vi "counter_sum.vi"(8 "error in":errorcluster) -> (0 "error IO":errorcluster, 1 "Number of Hours":dbl, 2 "Third Detector Sum":i64, 3 "First Detector Sum":i64)   [LabVIEW 2012]
uses:
  <vilib>/addons/database/Auxilliary.llb/DB Tools Parameter Info.ctl
  <vilib>/addons/database/Auxilliary.llb/DB Tools DataTypes.ctl
  <vilib>/addons/database/Auxilliary.llb/DB Tools Parameter Dir.ctl
  <vilib>/addons/database/Command.llb/Cmd Execute.vi
  <vilib>/addons/database/Recordset.llb/Rec Fetch Recordset Data (CR).vi
  <vilib>/addons/database/Recordset.llb/Rec Destroy - Command.vi
  <vilib>/addons/database/Command.llb/Cmd Delete.vi
  <vilib>/addons/database/Connection.llb/Conn Execute.vi
  <vilib>/addons/database/Recordset.llb/Rec Fetch Recordset Data (R).vi
  <vilib>/addons/database/Recordset.llb/Rec Destroy - Connection.vi
  <vilib>/addons/database/Command.llb/Cmd Set Parameter Value (C).vi
  <vilib>/addons/database/_DB Variant To Data/Database Variant To Data.xnode
  <vilib>/addons/database/NI_Database_API.lvlib
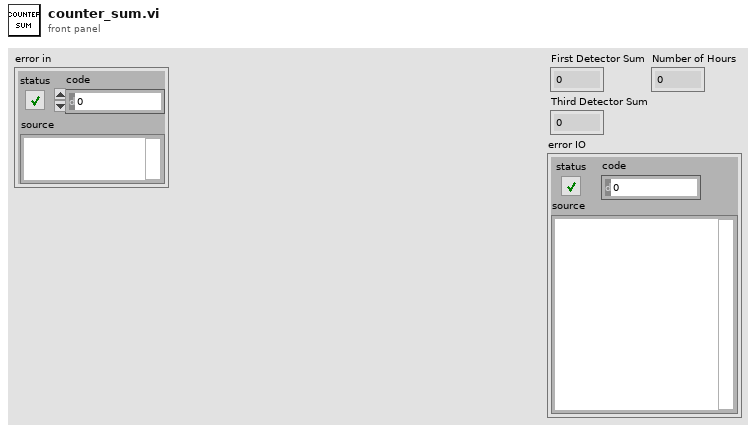
[diagram p1: front panel]
types:
  T1 = typedef "NI_Database_API.lvlib/DB Tools Parameter Info.ctl" = cluster{"parameter name":string, "type":T2, "direction":T3, "value":variant}
  T2 = typedef "NI_Database_API.lvlib/DB Tools DataTypes.ctl" = enum16{"String", "Long (I32)", "Single (SGL)", "Double (DBL)", "Date/Time", "Binary"}
  T3 = typedef "NI_Database_API.lvlib/DB Tools Parameter Dir.ctl" = enum32{"Input", "Output", "Input/Output", "Return Value"}
  T4 = typedef "NI_Database_API.lvlib/Conn ObjectReference.ctl" = refnum<k1>
  T5 = typedef "NI_Database_API.lvlib/Cmd ObjectReference.ctl" = refnum<k1>
  T6 = typedef "NI_Database_API.lvlib/Cmd-Rec Object Reference.ctl" = refnum<k1>
  T7 = typedef "NI_Database_API.lvlib/Rec ObjectReference.ctl" = refnum<k1>
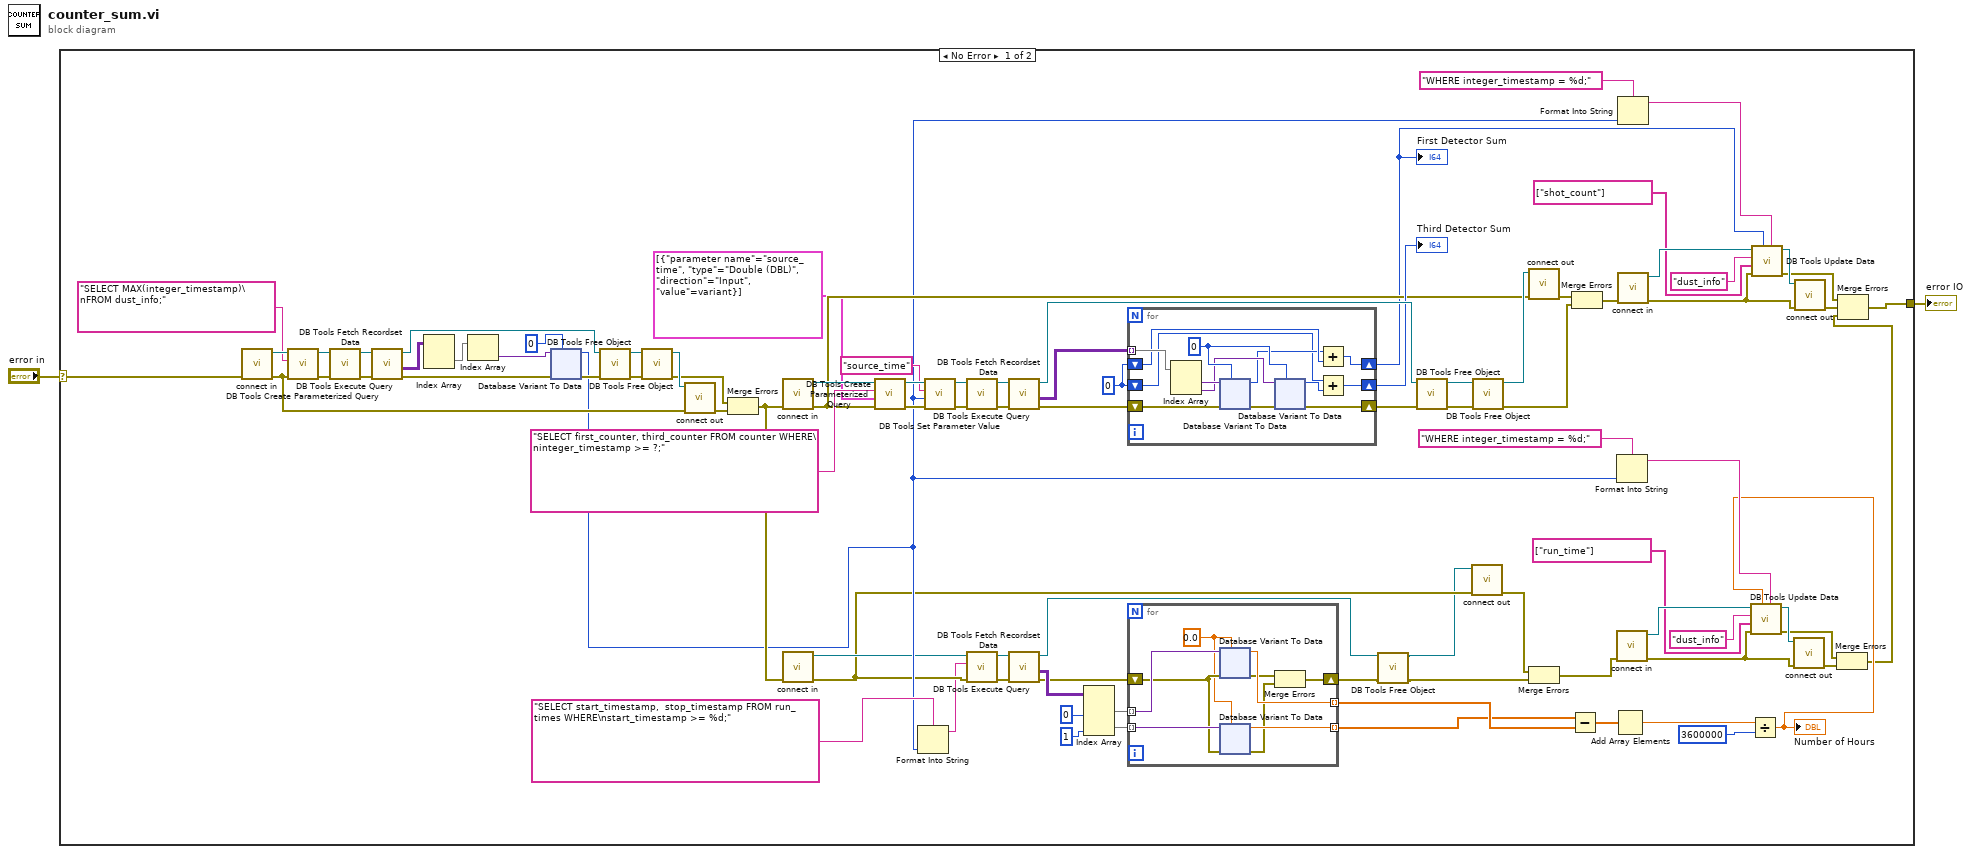
[diagram p0: block diagram]
diagram:
  n1 = case shown="No Error" "error in" {
    selector: "error in" -> [w92 w275]
    tunnel: [w49 w275] -> w1
    frame No Error {
      w60 = i64 0
      n2 = call "connect in.vi"("error in (no error)"=w92) -> ("error out"=w57:errorcluster, "Database Connection"=w91:T4)  [unwired: 6 in, 1 out]
      n3 = call <vilib>:"DB Tools Create Parameterized Query.vi"("error in (no error)"=w57, "SQL query"="SELECT MAX(integer_timestamp)\nFROM dust_info;", "connection reference"=w91) -> ("error out"=w88:errorcluster, "command reference"=w89:T5)  [unwired: 4 in, 1 out]
      n4 = call-poly <vilib>:"DB Tools Execute Query.vi"("error in (no error)"=w88, "command reference"=w89) -> ("error out"=w86:errorcluster, "command-recordset reference"=w87:T6)  [unwired: 6 in]
      n5 = call-poly <vilib>:"DB Tools Fetch Recordset Data.vi"("error in (no error)"=w86, "command-recordset reference"=w87) -> ("error out"=w78:errorcluster, "recordset data"=w82:variant[][], "command-recordset reference out"=w85:T6)  [unwired: 3 in]
      n6 = Index Array(array=w82) -> (element=w81:variant[])  [unwired: 2 in]
      n7 = Index Array(array=w81) -> (element=w80:variant)  [unwired: 1 in]
      n8 = xnode "Database Variant To Data"("database variant"=w80, "error in (no error)"=w78, "type"=i64 0) -> ("data"=w10:i64, "error out"=w77:errorcluster)
      n9 = call-poly <vilib>:"DB Tools Free Object.vi"("error in (no error)"=w77, "command-recordset reference"=w85) -> ("error out"=w83:errorcluster, "command reference"=w84:T5)  [unwired: 8 in]
      n10 = call-poly <vilib>:"DB Tools Free Object.vi"("error in (no error)"=w83, "command reference"=w84) -> ("error out"=w53:errorcluster, "connection reference"=w58:T4)  [unwired: 8 in]
      n11 = call "connect out.vi"("error in (no error)"=w57, "connection reference"=w58) -> ("error out"=w54:errorcluster)  [unwired: 9 in]
      n12 = Merge Errors(w53, w54) -> (w39:errorcluster)
      n13 = call "connect in.vi"("error in (no error)"=w39) -> ("error out"=w55:errorcluster, "Database Connection"=w56:T4)  [unwired: 6 in, 1 out]
      n14 = call "connect in.vi"("error in (no error)"=w39) -> ("error out"=w8:errorcluster, "Database Connection"=w9:T4)  [unwired: 6 in, 1 out]
      n15 = call <vilib>:"DB Tools Create Parameterized Query.vi"("error in (no error)"=w55, "parameters"=T1[] [{"parameter name"="source_time", "type"=enum."Double (DBL)", "direction"=enum."Input", "value"=variant}], "SQL query"="SELECT first_counter, third_counter FROM counter WHERE\ninteger_timestamp >= ?;", "connection reference"=w56) -> ("error out"=w74:errorcluster, "command reference"=w75:T5)  [unwired: 3 in, 1 out]
      n16 = Format Into String(format string="SELECT start_timestamp,  stop_timestamp FROM run_times WHERE\nstart_timestamp >= %d;" ("SQL query"), w10) -> (resulting string=w7:string)  [unwired: 2 in, 1 out]
      n17 = call-poly <vilib>:"DB Tools Set Parameter Value.vi"("error in (no error)"=w74, "value"=w10, "parameter index"="source_time" ("parameter name"), "command reference"=w75) -> ("error out"=w71:errorcluster, "command reference out"=w73:T5)  [unwired: 4 in]
      n18 = call-poly <vilib>:"DB Tools Execute Query.vi"("error in (no error)"=w71, "command reference"=w73) -> ("error out"=w70:errorcluster, "command-recordset reference"=w72:T6)  [unwired: 6 in]
      n19 = call-poly <vilib>:"DB Tools Execute Query.vi"("error in (no error)"=w8, "SQL query"=w7, "connection reference"=w9) -> ("error out"=w37:errorcluster, "recordset reference"=w36:T7)  [unwired: 5 in]
      n20 = call-poly <vilib>:"DB Tools Fetch Recordset Data.vi"("error in (no error)"=w70, "command-recordset reference"=w72) -> ("error out"=w62:errorcluster, "recordset data"=w69:variant[][], "command-recordset reference out"=w63:T6)  [unwired: 3 in]
      n21 = call-poly <vilib>:"DB Tools Fetch Recordset Data.vi"("error in (no error)"=w37, "recordset reference"=w36) -> ("error out"=w30:errorcluster, "recordset data"=w35:variant[][], "recordset reference out"=w6:T7)  [unwired: 3 in]
      n22 = Index Array(array=w35, index (col) #1=0 ("disabled index (col)"), index (col) #2=1 ("index (col)")) -> (element #1=w31:variant[], element #2=w32:variant[])  [unwired: 2 in]
      n23 = for {
        tunnel: w69 -> [w178] mode=indexing
        shift-right: [w174] -> w61
        shift-left: w62 -> [w176]
        shift-right: [w169] -> w45
        shift-left: w60 -> [w171]
        shift-right: [w166] -> w59
        shift-left: w60 -> [w167]
        w177 = i64 0
        n24 = Index Array(array=w178) -> (element #1=w173:variant, element #2=w172:variant)  [unwired: 2 in]
        n25 = xnode "Database Variant To Data"("database variant"=w173, "error in (no error)"=w176, "type"=w177) -> ("data"=w170:i64, "error out"=w175:errorcluster)
        n26 = xnode "Database Variant To Data"("database variant"=w172, "error in (no error)"=w175, "type"=w177) -> ("data"=w168:i64, "error out"=w174:errorcluster)
        n27 = Add(x=w170, y=w171) -> (x+y=w169:i64)
        n28 = Add(x=w167, y=w168) -> (x+y=w166:i64)
      }
      "First Detector Sum" <- w45
      "Third Detector Sum" <- w59
      n29 = for {
        tunnel: w31 -> [w101] mode=indexing
        tunnel: w32 -> [w100] mode=indexing
        tunnel: [w97] -> w12 mode=indexing
        tunnel: [w99] -> w13 mode=indexing
        shift-right: [w94] -> w5
        shift-left: w30 -> [w98]
        w93 = 0.0
        n30 = xnode "Database Variant To Data"("database variant"=w101, "error in (no error)"=w98, "type"=w93) -> ("data"=w99:dbl, "error out"=w96:errorcluster)
        n31 = xnode "Database Variant To Data"("database variant"=w100, "error in (no error)"=w98, "type"=w93) -> ("data"=w97:dbl, "error out"=w95:errorcluster)
        n32 = Merge Errors(w96, w95) -> (w94:errorcluster)
      }
      n33 = call-poly <vilib>:"DB Tools Free Object.vi"("error in (no error)"=w5, "recordset reference"=w6) -> ("error out"=w4:errorcluster, "connection reference"=w3:T4)  [unwired: 8 in]
      n34 = call-poly <vilib>:"DB Tools Free Object.vi"("error in (no error)"=w61, "command-recordset reference"=w63) -> ("error out"=w66:errorcluster, "command reference"=w68:T5)  [unwired: 8 in]
      n35 = call "connect out.vi"("error in (no error)"=w8, "connection reference"=w3) -> ("error out"=w26:errorcluster)  [unwired: 9 in]
      n36 = call-poly <vilib>:"DB Tools Free Object.vi"("error in (no error)"=w66, "command reference"=w68) -> ("error out"=w64:errorcluster, "connection reference"=w67:T4)  [unwired: 8 in]
      n37 = call "connect out.vi"("error in (no error)"=w55, "connection reference"=w67) -> ("error out"=w65:errorcluster)  [unwired: 9 in]
      n38 = Merge Errors(w26, w4) -> (w15:errorcluster)
      n39 = Subtract(x=w12, y=w13) -> (x-y=w29:dbl[])
      n40 = Merge Errors(w65, w64) -> (w52:errorcluster)
      n41 = Add Array Elements(numeric array=w29) -> (sum=w28:dbl)
      n42 = Format Into String(format string="WHERE integer_timestamp = %d;" ("condition"), w10) -> (resulting string=w20:string)  [unwired: 2 in, 1 out]
      n43 = call "connect in.vi"("error in (no error)"=w15) -> ("error out"=w24:errorcluster, "Database Connection"=w25:T4)  [unwired: 6 in, 1 out]
      n44 = Format Into String(format string="WHERE integer_timestamp = %d;" ("condition"), w10) -> (resulting string=w43:string)  [unwired: 2 in, 1 out]
      n45 = call "connect in.vi"("error in (no error)"=w52) -> ("error out"=w50:errorcluster, "Database Connection"=w51:T4)  [unwired: 6 in, 1 out]
      n46 = Divide(x=w28, y=i64 3600000) -> (x/y=w16:dbl)
      "Number of Hours" <- w16
      n47 = call <vilib>:"DB Tools Update Data.vi"("condition"=w20, "data"=w16, "error in (no error)"=w24, "columns"=string[] ["run_time"], "table"="dust_info", "connection reference"=w25) -> ("error out"=w21:errorcluster, "connection reference out"=w22:T4)  [unwired: 4 in]
      n48 = call <vilib>:"DB Tools Update Data.vi"("condition"=w43, "data"=w45, "error in (no error)"=w50, "columns"=string[] ["shot_count"], "table"="dust_info", "connection reference"=w51) -> ("error out"=w46:errorcluster, "connection reference out"=w47:T4)  [unwired: 4 in]
      n49 = call "connect out.vi"("error in (no error)"=w24, "connection reference"=w22) -> ("error out"=w23:errorcluster)  [unwired: 9 in]
      n50 = call "connect out.vi"("error in (no error)"=w50, "connection reference"=w47) -> ("error out"=w48:errorcluster)  [unwired: 9 in]
      n51 = Merge Errors(w21, w23) -> (w14:errorcluster)
      n52 = Merge Errors(w46, w48, w14) -> (w49:errorcluster)
    }
    frame Error {
    }
  }
  "error IO" <- w1
